vi "Ramsete Controller.vi"(8 "Turing Parameters":cluster{"b":dbl, "zeta":dbl}={"b"=2.0, "zeta"=0.7}, 9 "Velocity Ref":T1 {"Angular Velocity Ref" format="%#_13g"; "Linear Velocity Ref" format="%#_13g"}, 10 "Pose Ref":T2, 11 "Current Pose":T2) -> (2 "Angular Velocity":dbl, 3 "Linear Velocity":dbl)   [LabVIEW 2019]
uses:
  Geometry/Typedef/Pose2d.ctl
  Geometry/Typedef/Translation2d.ctl
  Geometry/Typedef/Rotation2d.ctl
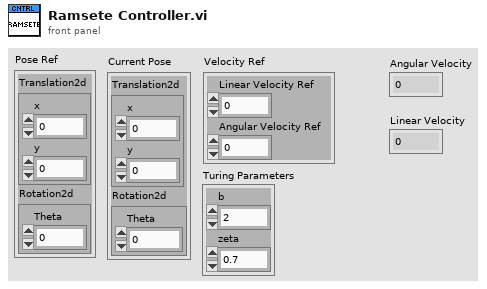
[diagram p1: front panel]
types:
  T1 = cluster{"Linear Velocity Ref":dbl, "Angular Velocity Ref":dbl}
  T2 = typedef "Pose2d.ctl" = cluster{"Translation2d":T3, "Rotation2d":T4}
  T3 = typedef "Translation2d.ctl" = cluster{"x":dbl, "y":dbl}
  T4 = typedef "Rotation2d.ctl" = cluster{"Theta":dbl}
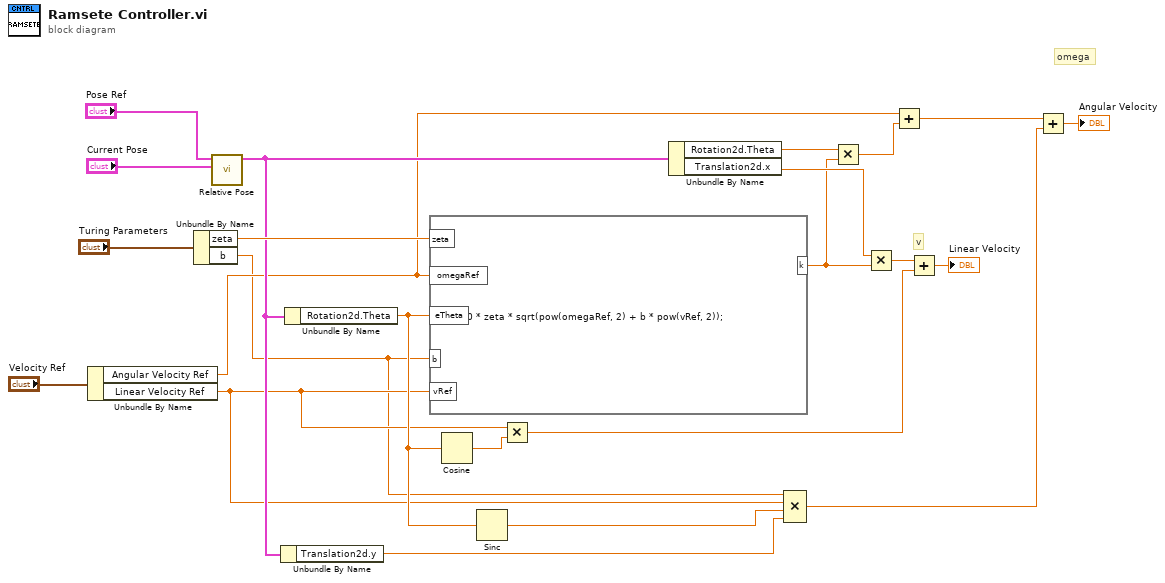
[diagram p0: block diagram]
diagram:
  # "omega"
  # "v"
  n1 = Unbundle By Name("Velocity Ref") -> ("Angular Velocity Ref"=w4:dbl, "Linear Velocity Ref"=w2:dbl)
  n2 = Unbundle By Name("Turing Parameters") -> ("zeta"=w23:dbl, "b"=w1:dbl)
  n3 = call "Relative Pose.vi"("Final"="Current Pose", "Initial"="Pose Ref") -> ("Relative Pose"=w14:T2)  [unwired: 9 in]
  n4 = Unbundle By Name(w14) -> ("Translation2d.y"=w15:dbl)
  n5 = Unbundle By Name(w14) -> ("Rotation2d.Theta"=w16:dbl)
  n6 = formula code="k = 2.0 * zeta * sqrt(pow(omegaRef, 2) + b * pow(vRef, 2));"("zeta"=w23, "omegaRef"=w4, "eTheta"=w16, "b"=w1, "vRef"=w2) -> ("k"=w3:dbl)
  n7 = Cosine(x=w16) -> (cos(x)=w8:dbl)
  n8 = Sinc(1:w16) -> (0:w17:dbl)
  n9 = Multiply(x=w2, y=w8) -> (x*y=w9:dbl)
  n10 = Unbundle By Name(w14) -> ("Rotation2d.Theta"=w12:dbl, "Translation2d.x"=w10:dbl)
  n11 = Compound Arithmetic op=MULTIPLY(w1, w2, w17, w15) -> (w19:dbl)
  n12 = Multiply(x=w12, y=w3) -> (x*y=w13:dbl)
  n13 = Multiply(x=w10, y=w3) -> (x*y=w11:dbl)
  n14 = Add(x=w4, y=w13) -> (x+y=w18:dbl)
  n15 = Add(x=w11, y=w9) -> (x+y=→"Linear Velocity":dbl)
  n16 = Add(x=w18, y=w19) -> (x+y=→"Angular Velocity":dbl)
